vi "StripLeadingTrailingSpaces.vi"(10 "StringIn":string) -> (2 "NoLeadingOrTrailingSpaces":string)   [LabVIEW 2018]
panel:
  # "Copyright © 2011 Epimedia, Inc. All Rights Reserved.\n\nThe Epimedia Application Library is Copyright © 2009-2011 Epimedia, Inc. \nAll Rights Reserved. Used under license."
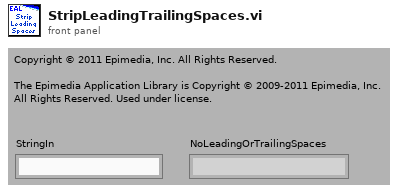
[diagram p1: front panel]
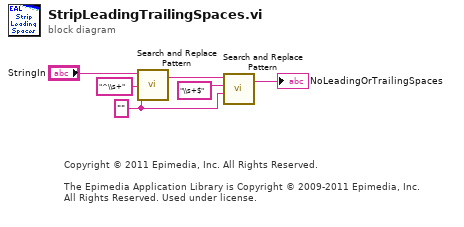
[diagram p0: block diagram]
diagram:
  w2 = "" ("replace string (\"\")")
  # "Copyright © 2011 Epimedia, Inc. All Rights Reserved.\n\nThe Epimedia Application Library is Copyright © 2009-2011 Epimedia, Inc. \nAll Rights Reserved. Used under license."
  n1 = call <vilib>:"Search and Replace Pattern.vi"("string"="StringIn", "regular expression (\"\")"="^\\s+" ("regular expression (\"\")"), "replace string (\"\")"=w2) -> ("result string"=w4:string)  [unwired: 2 in, 1 out]
  n2 = call <vilib>:"Search and Replace Pattern.vi"("string"=w4, "regular expression (\"\")"="\\s+$" ("regular expression (\"\")"), "replace string (\"\")"=w2) -> ("result string"=→"NoLeadingOrTrailingSpaces":string)  [unwired: 2 in, 1 out]
